vi "Flatten Tags to JSON List.vi"(8 "error in (no error)":errorcluster, 10 "Tag Names (all)":string[](array[string])) -> (0 "error out":errorcluster, 2 "JSON List out":string)   [LabVIEW 2020, in "Tag Engine.lvlib"]
doc: "Create a JSON array of Tag configurations from a list of Tags.\n\nIf the input list of Tag Names is empty, all Tags will be used to generate the JSON array."
uses:
  Tag Engine.lvlib
  Tag/Tag.lvclass
  <vilib>/JDP Science/JSONtext/JSONtext.lvlib
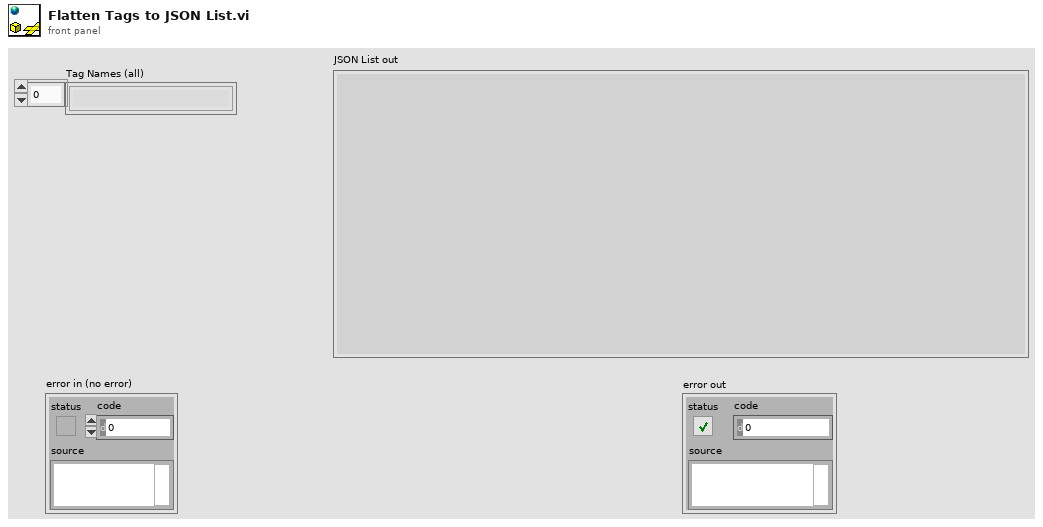
[diagram p1: front panel]
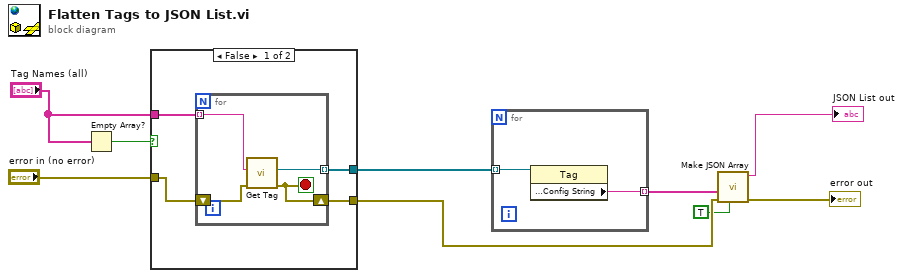
[diagram p0: block diagram]
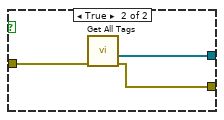
[diagram p2: hidden frame]
diagram:
  n1 = Empty Array?(array="Tag Names (all)") -> (empty?=w9:bool)
  n2 = case shown="False" w9 {
    tunnel: "error in (no error)" -> [w11 w20]
    tunnel: [w12 w19] -> w6
    tunnel: "Tag Names (all)" -> [w13 _]
    tunnel: [w10 w18] -> w3
    frame False {
      n3 = for {
        tunnel: w13 -> [w17] mode=indexing
        tunnel: [w16] -> w12 mode=indexing
        shift-right: [w14] -> w10
        shift-left: w11 -> [w15]
        stop <- w14 stop-if-true
        n4 = call "Get Tag.vi"("error in (no error)"=w15, "Name"=w17) -> ("error out"=w14:errorcluster, "Tag Ref out"=w16:refnum<data-value>)  [unwired: 7 in, 1 out]
      }
    }
    frame True {
      n5 = call "Get All Tags.vi"("error in (no error)"=w20) -> ("error out"=w18:errorcluster, "Tag Refs"=w19:refnum<data-value>[])  [unwired: 8 in, 1 out]
    }
  }
  n6 = for {
    tunnel: w6 -> [w22] mode=indexing
    tunnel: [w21] -> w5 mode=indexing
    n7 = property class="Tag"(reference=w22) -> ("Properties:Config String"=w21:string)  [unwired: 1 in, 2 out]
  }
  n8 = call <vilib>:"Make JSON Array.vi"("Pretty Print?"=TRUE, "error in (no error)"=w3, "JSON Elements"=w5) -> ("error out"=→"error out":errorcluster, "<JSON>"=→"JSON List out":string)  [unwired: 7 in]
